vi "CR-扫码枪.vi"(8 "error in (no error)":errorcluster caption="错误输入（无错误）", 11 "名称或相对路径":string="Template Program") -> (0 "error in (no error) 2":errorcluster caption="错误输入（无错误）")   [LabVIEW 2017]
uses:
  Picture/SaveButtom.ctl
  Global System.vi
  <vilib>/Utility/xml.llb/Write to XML File(string).vi
panel:
  out "添加的路径":path
  in  "刷新":bool
  in  "测试按钮":bool
  in  "保存按钮":bool
  in  "Main":enum32{"条码获取", "测试效果 "}(tab)
  in  "扫码枪基础参数":T1 caption="参数界面"
  in  "扫码枪参数":T2={"IsNorImage"=TRUE, "Exposure Values"=100289, "ImagePath"=path "C:/Users/hedongpo/Desktop/514-hdp/Alignment Assemble System/Test Picture/B/3.bmp", "数据输出"="", "结果显示"=FALSE} caption="参数界面" {"Exposure Values" scale=0.0..200000.0}
  out "路径输出":path
  in  "Vision Paramter Save Buttom":T3
  out "system time":string
  in  "取消按钮":bool
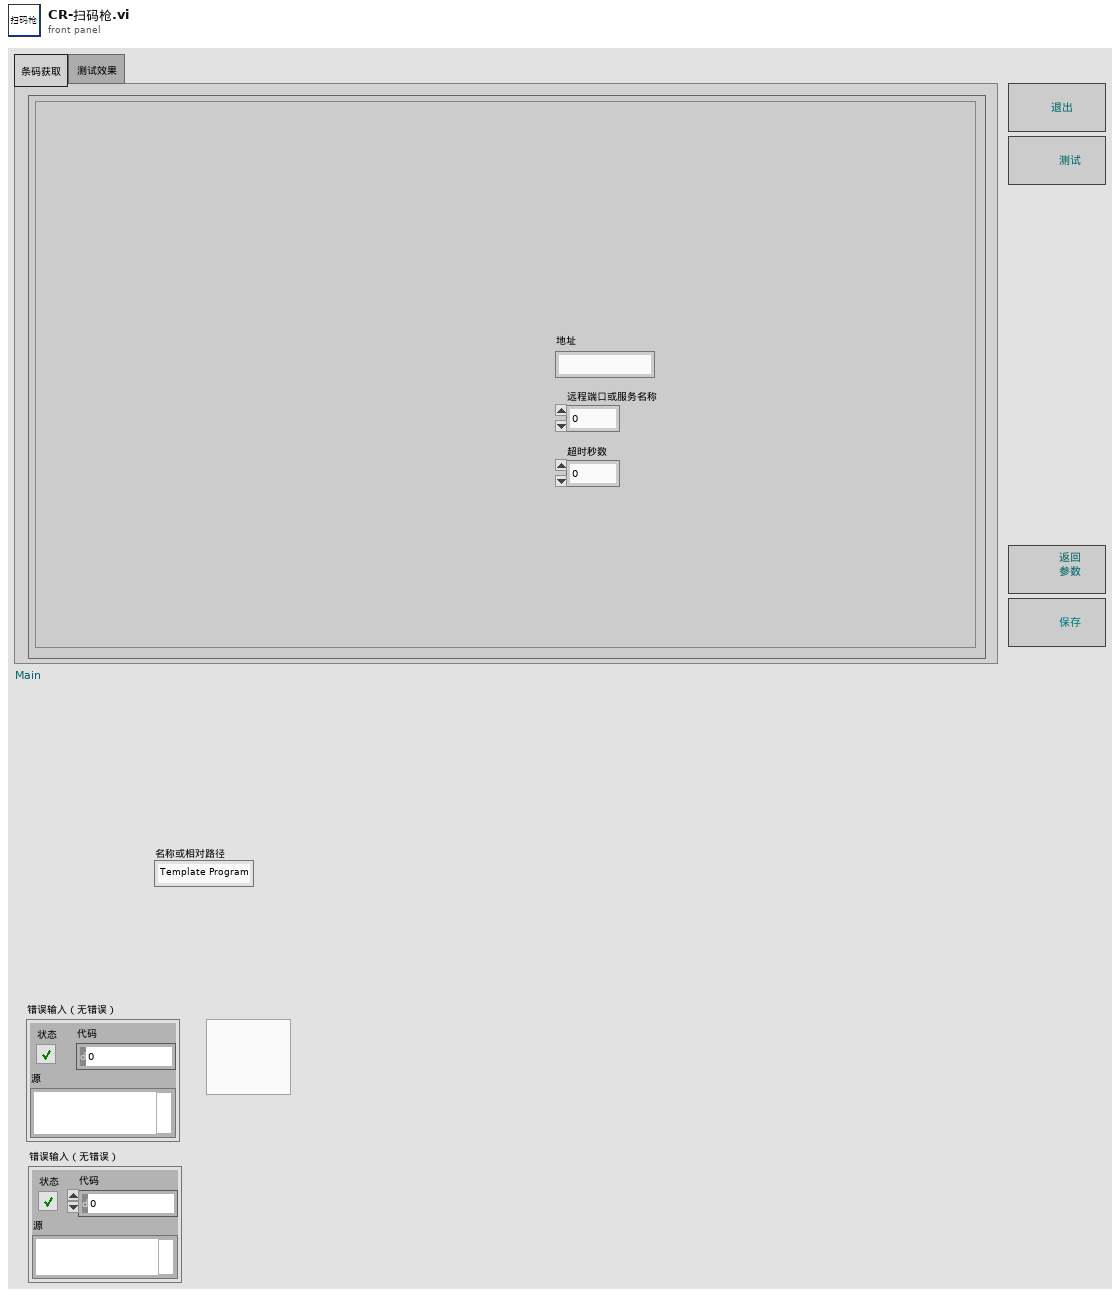
[diagram p1: front panel]
types:
  T1 = cluster{"地址":string, "远程端口或服务名称":u16, "超时秒数":dbl}
  T2 = cluster{"IsNorImage":bool, "Exposure Values":u32, "ImagePath":path, "数据输出":string, "结果显示":bool}
  T3 = typedef "SaveButtom.ctl" = bool
  T4 = cluster{"index":i32, "this vi":refnum<vi>, "error out":errorcluster}
  T5 = cluster{"master data":string, "priority":u16, "secondary data":string[]}
  T6 = cluster{"case name":string[], "queue array":refnum<queue>[]}
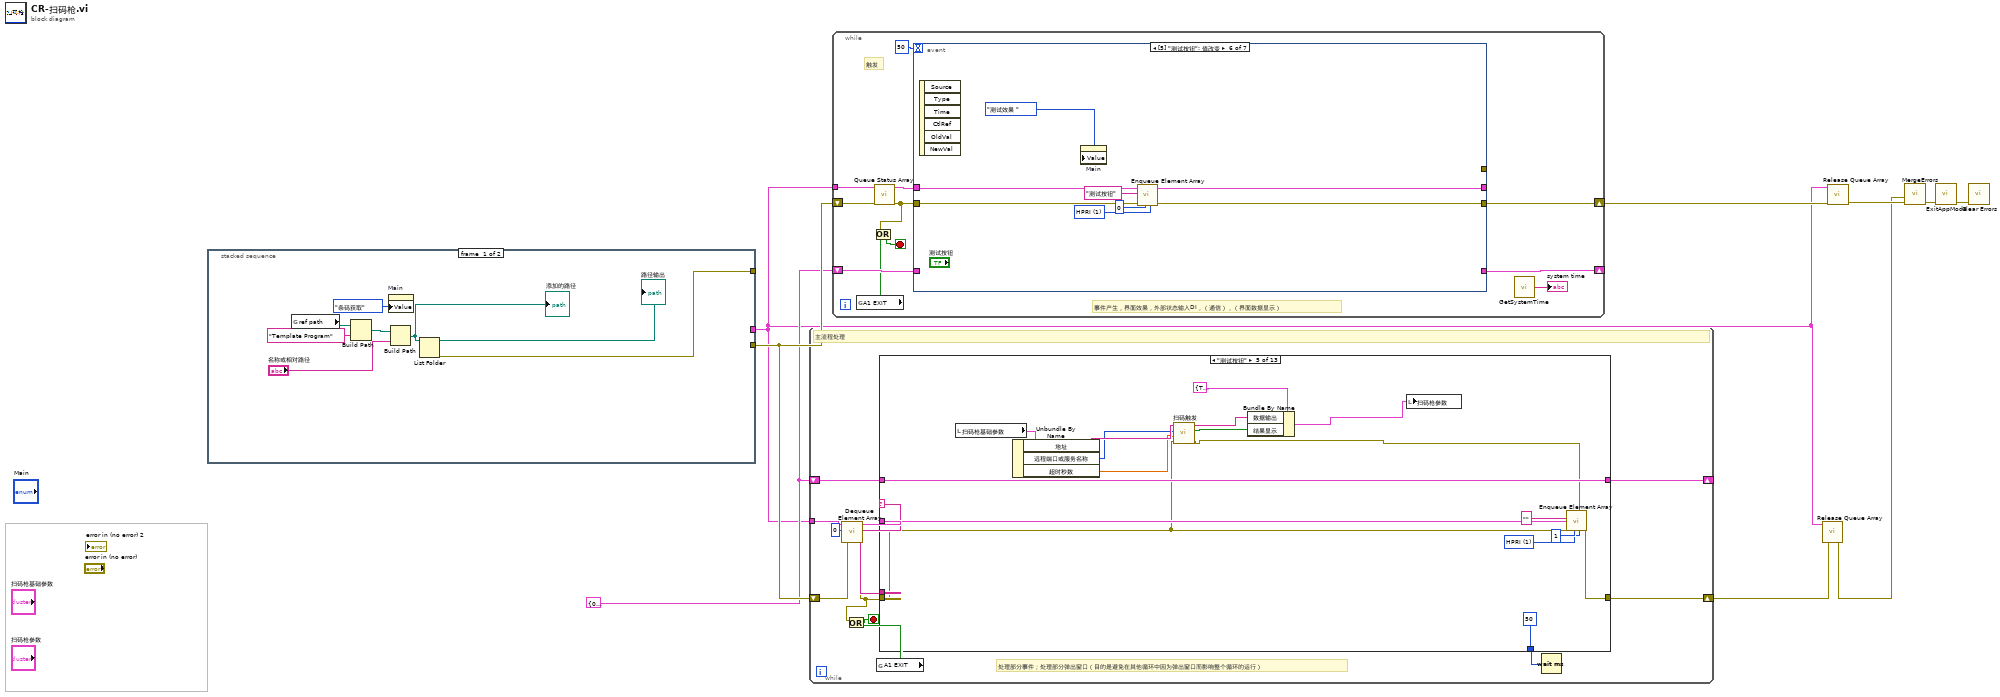
[diagram p0: block diagram]
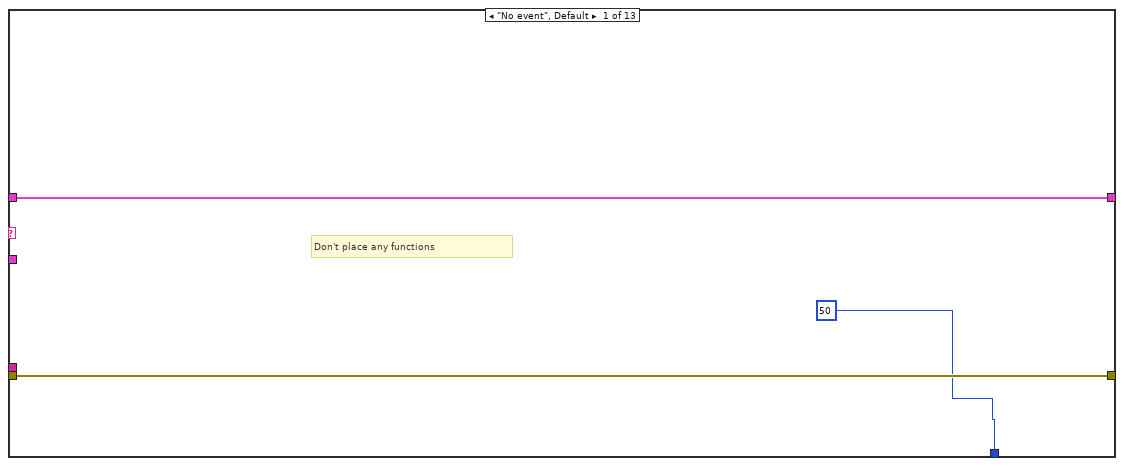
[diagram p2: hidden frame]
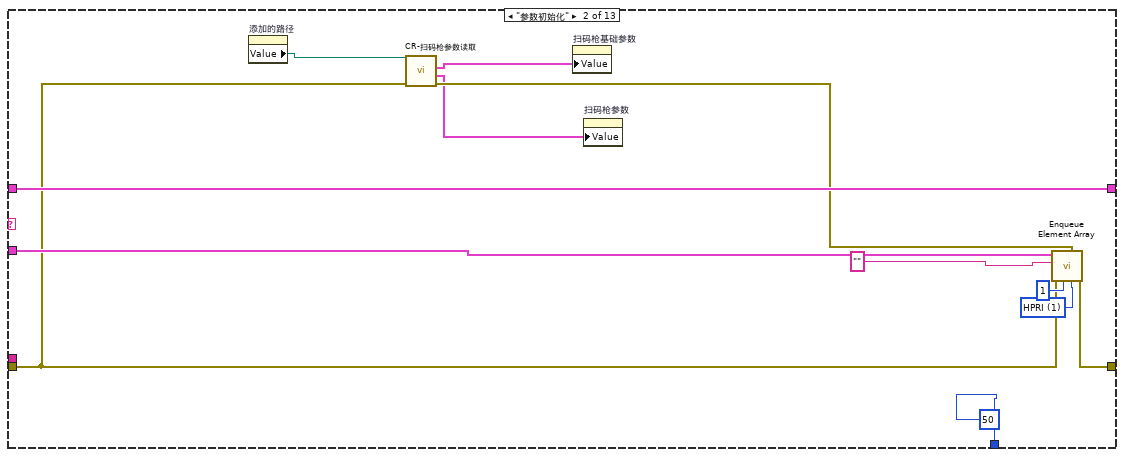
[diagram p3: hidden frame]
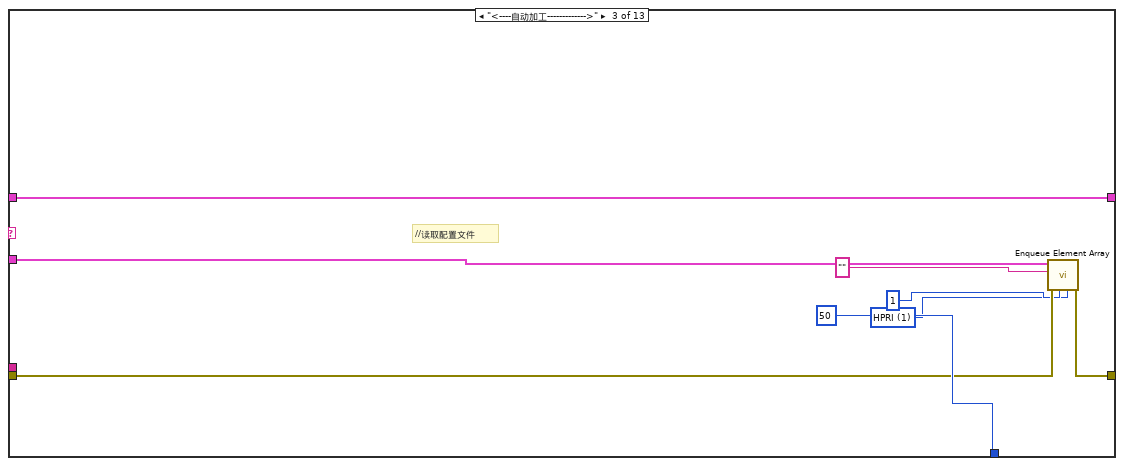
[diagram p4: hidden frame]
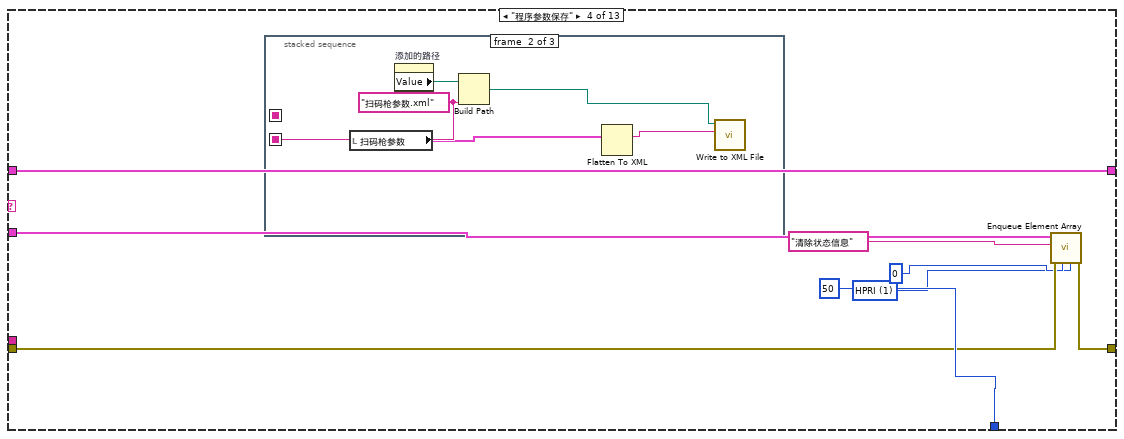
[diagram p5: hidden frame]
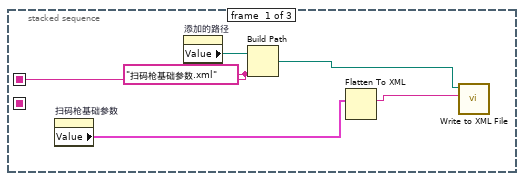
[diagram p6: hidden frame]
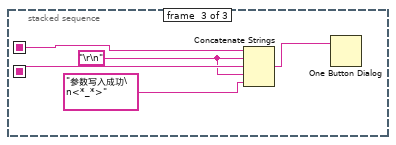
[diagram p7: hidden frame]
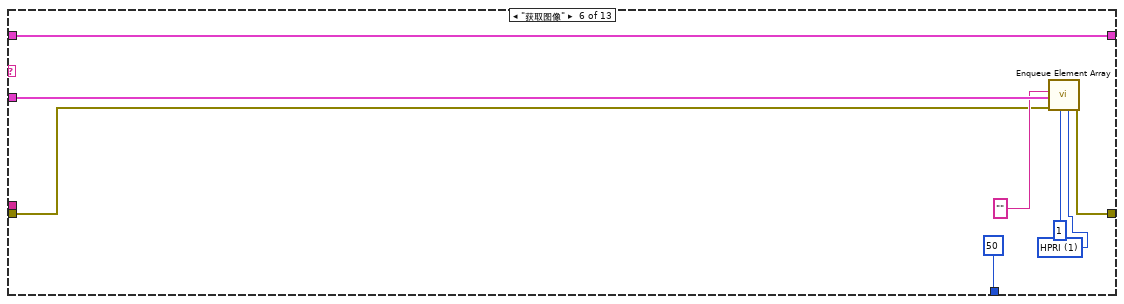
[diagram p8: hidden frame]
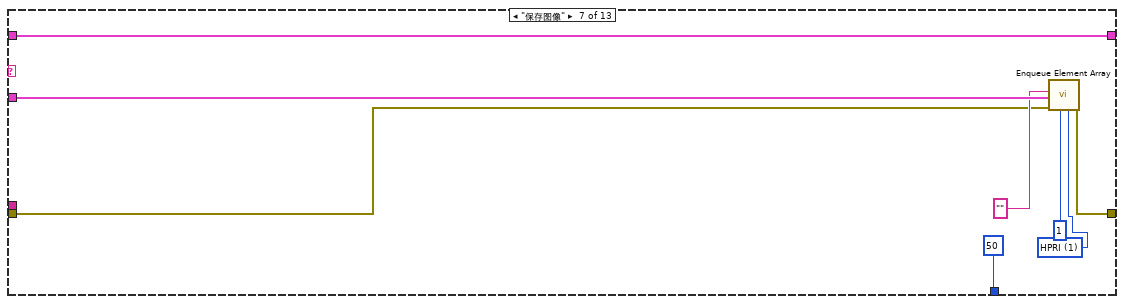
[diagram p9: hidden frame]
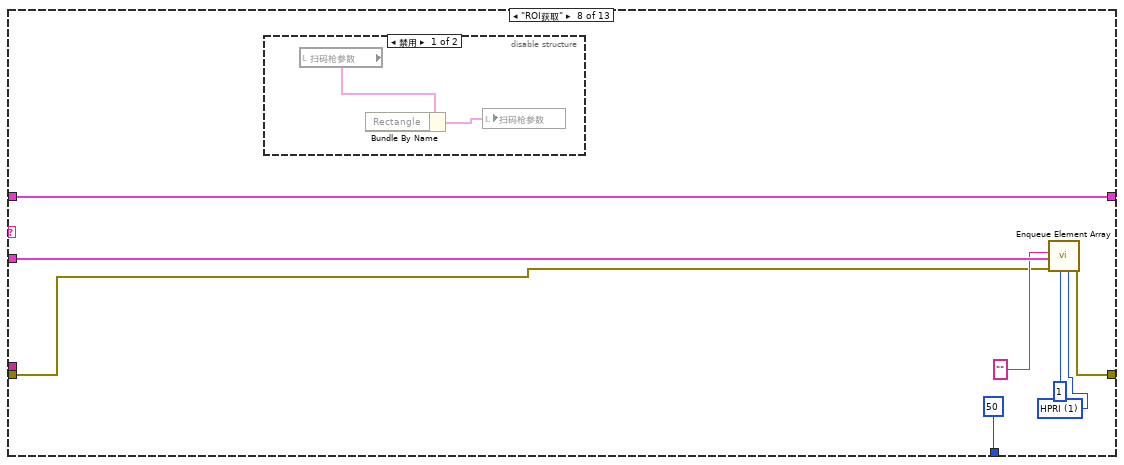
[diagram p10: hidden frame]
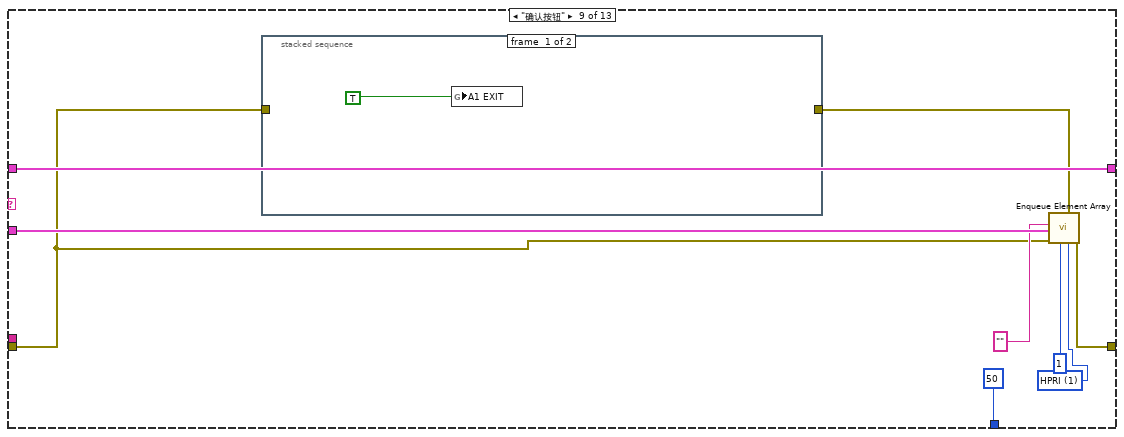
[diagram p12: hidden frame]
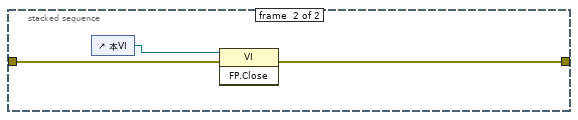
[diagram p13: hidden frame]
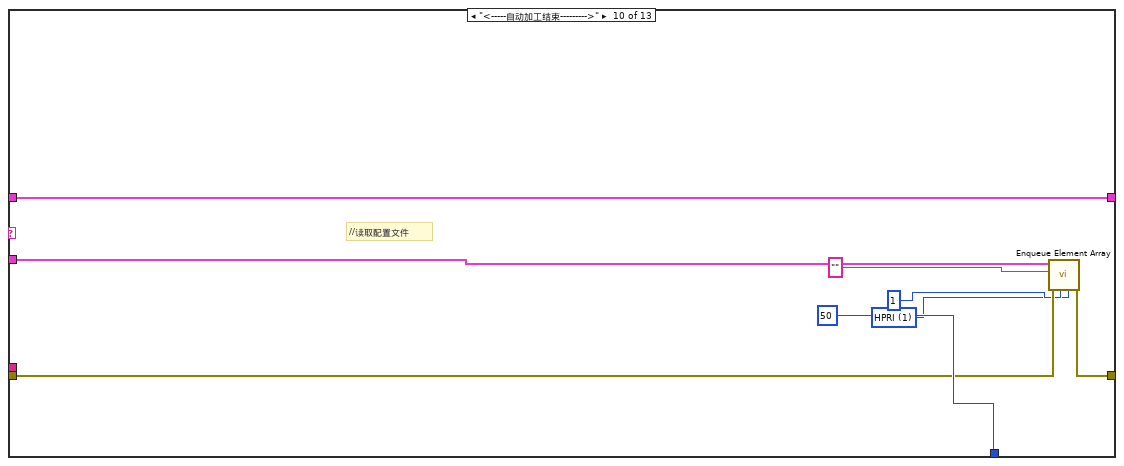
[diagram p14: hidden frame]
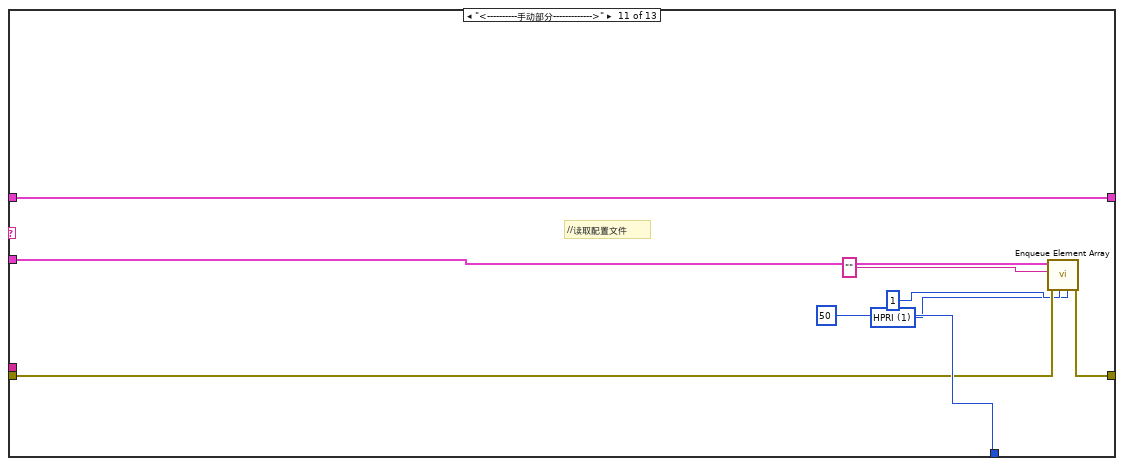
[diagram p15: hidden frame]
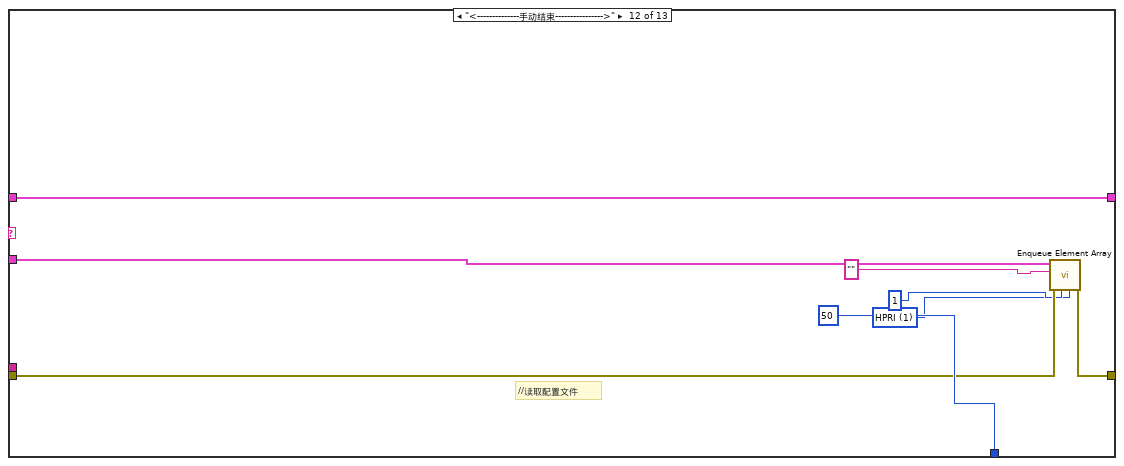
[diagram p16: hidden frame]
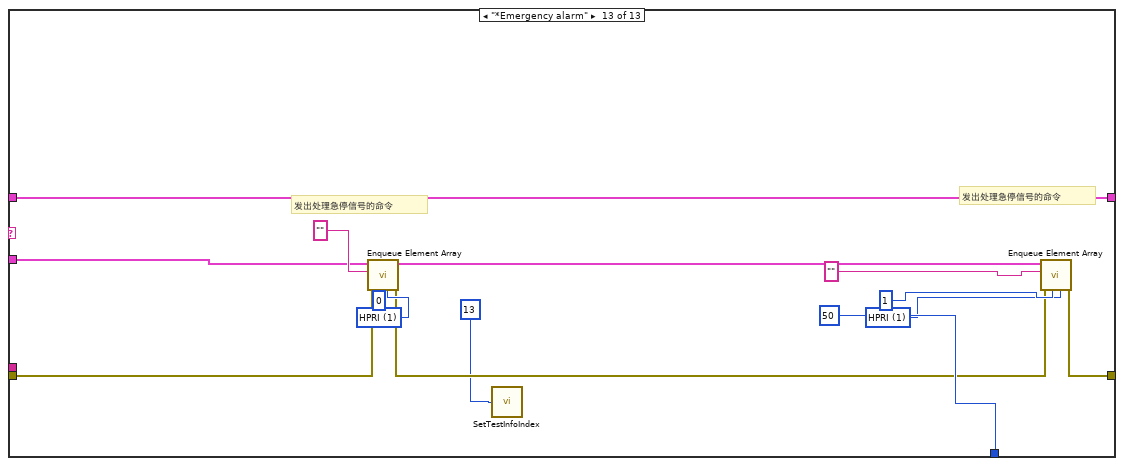
[diagram p17: hidden frame]
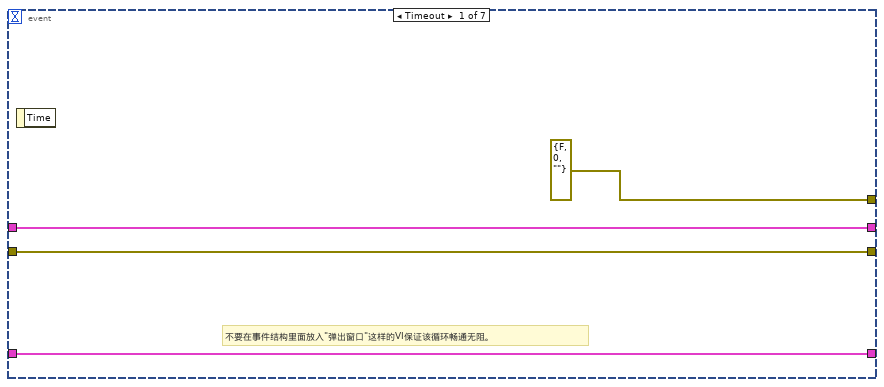
[diagram p18: hidden frame]
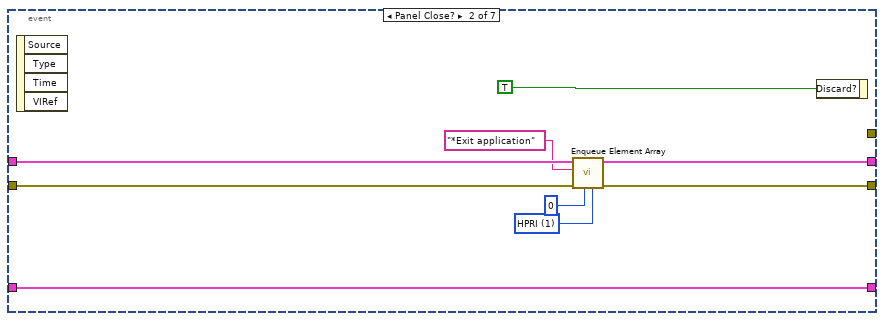
[diagram p19: hidden frame]
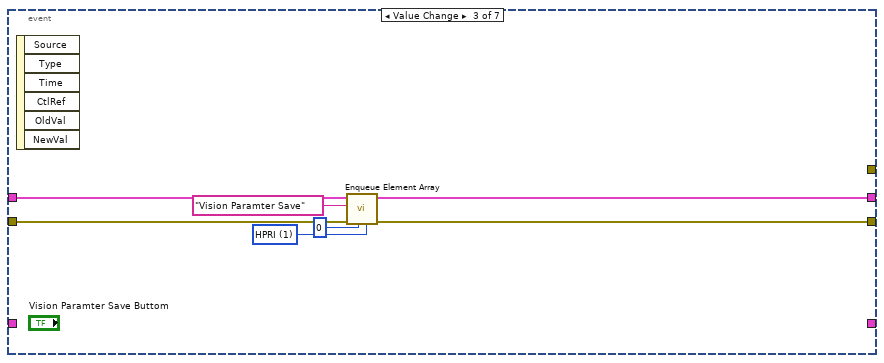
[diagram p20: hidden frame]
diagram:
  w4 = T4 {"index"=0, "this vi"=refnum, "error out"={"status"=FALSE, "code"=0, "source"=""}} ("parameter buffer")
  n1 = stacked-sequence {
    tunnel: [w15 _] -> _
    tunnel: [_ w19] -> w5
    tunnel: [_ w18] -> w1
    frame #0 {
      n2 = global read "Global System.vi" "ref path"() -> (w13:path)
      n3 = Build Path(base path=w13, name or relative path="Template Program" ("名称或相对路径")) -> (appended path=w11:path)
      n4 = property on="Main" class="TabCtl (严格)"("Value"=enum32{"条码获取", "测试效果 "}."条码获取" ("Main")) -> ()  [unwired: 2 in, 2 out]
      n5 = Build Path(base path=w11, name or relative path="名称或相对路径") -> (appended path=w17:path)
      "添加的路径" <- w17
      n6 = List Folder(path=w17) -> (path out=→"路径输出":path, error out=w15:errorcluster)  [unwired: 3 in, 2 out]
    }
    frame #1 {
      w27 = string[] ["comm queue1", "data queue 11", "data queue 12", "data queue 13", "data queue 14"]  # queue name
      w28 = 4  # queue num
      w29 = T5 {"master data"="", "priority"=0, "secondary data"=[]}  # element data type
      n7 = call "Obtain Queue Array.vi"("queue name"=w27, "element data type"=w29, "queue num"=w28) -> ("error out"=w23:errorcluster, "queue out"=w24:T6)  [unwired: 2 in, 1 out]
      n8 = call "Enqueue Element Array.vi"("queue index"=0, "error in"=w23, "master data"="参数初始化", "queue in"=w24) -> ("error out"=w22:errorcluster, "queue out"=w21:T6)  [unwired: 6 in]
      n9 = disable-structure shown="启用" {
        disable-tunnel: w22 -> [w35 w36]
        disable-tunnel: w21 -> [w34 w37]
        disable-tunnel: "Loading Variable" ("master data") -> [w33 _]
        disable-tunnel: [w31 w36] -> w19
        disable-tunnel: [w30 w37] -> w18
        frame Disabled {
          n10 = call "Enqueue Element Array.vi"("queue index"=12, "error in"=w35, "master data"=w33, "queue in"=w34) -> ("error out"=w31:errorcluster, "queue out"=w30:T6)  [unwired: 6 in]
        }
        frame Enabled {
        }
      }
    }
  }
  n11 = while {
    shift-right: [w50] -> w3
    shift-left: w5 -> [w41]
    shift-right: [w47] -> _
    shift-left: w4 -> [w48]
    tunnel: w1 -> [w43]
    stop <- w38 stop-if-true
    # "处理部分事件；处理部分弹出窗口（目的是避免在其他循环中因为弹出窗口而影响整个循环的运行）"
    # "主流程处理"
    n12 = call "Dequeue Element Array.vi"("queue in"=w43, "queue index"=0, "error in"=w41) -> ("queue out"=w46:T6, "master data"=w45:string, "secondary data"=w44:string[], "error out"=w40:errorcluster)  [unwired: 2 in, 1 out]
    n13 = global read "Global System.vi" "A1 EXIT"() -> (w39:bool)
    n14 = Or(x=w40, y=w39) -> (x .or. y?=w38:bool)
    n15 = case shown="\"测试按钮\"" w45 {
      tunnel: w46 -> [_ w64 w72 w74 w112 w120 w128 w136 w147 w159 w167 w175 w181]
      tunnel: w40 -> [w52 w57 w68 w78 w106 w114 w122 w130 w141 w155 w163 w171 w178]
      tunnel: [w52 w63 w71 w80 w111 w119 w127 w135 w146 w158 w166 w174 w189] -> w50
      tunnel: [50 50 50 50 50 50 50 50 50 50 50 50 50] -> w49
      tunnel: w48 -> [w53 w59 w69 w75 w107 w115 w123 w131 w142 w156 w164 w172 w187]
      tunnel: [w53 w59 w69 w75 w107 w115 w123 w131 w142 w156 w164 w172 w187] -> w47
      tunnel: w44 -> [_ _ _ _ _ _ _ _ _ _ _ _ _]
      frame "No event", Default {
        # "Don't place any functions"
      }
      frame "参数初始化" {
        w60 = u16 1 items=["HPRI"=1, "LPRI"=0] ("priority")
        n16 = property on="添加的路径" class="Path"() -> ("Value"=w58:path)  [unwired: 2 in, 2 out]
        n17 = call "CR-扫码枪参数读取.vi"("error in (no error)"=w57, "基路径"=w58) -> ("error out"=w56:errorcluster, "扫码枪参数"=w55:T2, "扫码枪基础参数"=w54:T1)  [unwired: 6 in]
        n18 = property on="扫码枪基础参数" class="Clust (严格)"("Value"=w54) -> ()  [unwired: 2 in, 2 out]
        n19 = property on="扫码枪参数" class="Clust (严格)"("Value"=w55) -> ()  [unwired: 2 in, 2 out]
        n20 = call "Enqueue Element Array.vi"("priority"=w60, "device error in"=w56, "queue index"=1, "error in"=w57, "master data"="" ("Element 1"), "queue in"=w64) -> ("error out"=w63:errorcluster)  [unwired: 4 in, 1 out]
      }
      frame "<----自动加工------------->" {
        w66 = u16 1 items=["HPRI"=1, "LPRI"=0] ("priority")
        # "//读取配置文件"
        n21 = call "Enqueue Element Array.vi"("priority"=w66, "queue index"=1, "error in"=w68, "master data"="" ("Element 1"), "queue in"=w72) -> ("error out"=w71:errorcluster)  [unwired: 5 in, 1 out]
      }
      frame "程序参数保存" {
        w76 = u16 1 items=["HPRI"=1, "LPRI"=0] ("priority")
        n22 = stacked-sequence {
          seq-local: [w82 _ _] -> [_ _ w95]
          seq-local: [_ w91 _] -> [_ _ w93]
          frame #0 {
            w82 = "扫码枪基础参数.xml" ("名称或相对路径")
            n23 = property on="扫码枪基础参数" class="Clust (严格)"() -> ("Value"=w85:T1)  [unwired: 2 in, 2 out]
            n24 = property on="添加的路径" class="Path"() -> ("Value"=w86:path)  [unwired: 2 in, 2 out]
            n25 = Build Path(base path=w86, name or relative path=w82) -> (appended path=w83:path)
            n26 = Flatten To XML(anything=w85) -> (xml string=w84:string)
            n27 = call-poly <vilib>:"Write to XML File.vi"("XML Input"=w84, "XML File Path"=w83) -> ()  [unwired: 7 in, 3 out]
          }
          frame #1 {
            w91 = "扫码枪参数.xml" ("名称或相对路径")
            n28 = local read "扫码枪参数"() -> (w87:T2)
            n29 = property on="添加的路径" class="Path"() -> ("Value"=w90:path)  [unwired: 2 in, 2 out]
            n30 = Build Path(base path=w90, name or relative path=w91) -> (appended path=w88:path)
            n31 = Flatten To XML(anything=w87) -> (xml string=w89:string)
            n32 = call-poly <vilib>:"Write to XML File.vi"("XML Input"=w89, "XML File Path"=w88) -> ()  [unwired: 7 in, 3 out]
          }
          frame #2 {
            w92 = "\r\n"
            n33 = Concatenate Strings(w95, w92, w93, w92, "参数写入成功\n<*_*>" ("消息")) -> (w94:string)
            n34 = One Button Dialog(message=w94) -> ()  [unwired: 1 in, 1 out]
          }
        }
        n35 = call "Enqueue Element Array.vi"("priority"=w76, "queue index"=0, "error in"=w78, "master data"="清除状态信息" ("Element 1"), "queue in"=w74) -> ("error out"=w80:errorcluster)  [unwired: 5 in, 1 out]
      }
      frame "测试按钮" {
        w108 = u16 1 items=["HPRI"=1, "LPRI"=0] ("priority")
        n36 = local read "扫码枪基础参数"() -> (w104:T1)
        n37 = Unbundle By Name(w104) -> ("地址"=w103:string, "远程端口或服务名称"=w102:u16, "超时秒数"=w97:dbl)
        n38 = call "扫码触发.vi"("error in (no error)"=w106, "超时秒数"=w97, "远程端口或服务名称"=w102, "地址"=w103) -> ("error out 2"=w105:errorcluster, "结果"=w100:bool, "数据输出"=w101:string)  [unwired: 5 in]
        n39 = Bundle By Name(cluster=T2 {"IsNorImage"=TRUE, "Exposure Values"=100289, "ImagePath"=path "C:/Users/hedongpo/Desktop/514-hdp/Alignment Assemble System/Test Picture/B/3.bmp", "数据输出"="", "结果显示"=FALSE} ("扫码枪参数"), "数据输出"=w101, "结果显示"=w100) -> (w98:T2)
        n40 = local write "扫码枪参数"(w98) -> ()
        n41 = call "Enqueue Element Array.vi"("priority"=w108, "device error in"=w105, "queue index"=1, "error in"=w106, "master data"="" ("Element 1"), "queue in"=w112) -> ("error out"=w111:errorcluster)  [unwired: 4 in, 1 out]
      }
      frame "获取图像" {
        w116 = u16 1 items=["HPRI"=1, "LPRI"=0] ("priority")
        n42 = call "Enqueue Element Array.vi"("priority"=w116, "queue index"=1, "error in"=w114, "master data"="" ("Element 1"), "queue in"=w120) -> ("error out"=w119:errorcluster)  [unwired: 5 in, 1 out]
      }
      frame "保存图像" {
        w124 = u16 1 items=["HPRI"=1, "LPRI"=0] ("priority")
        n43 = call "Enqueue Element Array.vi"("priority"=w124, "queue index"=1, "error in"=w122, "master data"="" ("Element 1"), "queue in"=w128) -> ("error out"=w127:errorcluster)  [unwired: 5 in, 1 out]
      }
      frame "ROI获取" {
        w132 = u16 1 items=["HPRI"=1, "LPRI"=0] ("priority")
        n44 = disable-structure shown="禁用" {
          frame Disabled {
            n45 = local read "扫码枪参数"() -> (w139:T2)
            n46 = Bundle By Name(cluster=w139) -> (w138:T2)  [unwired: 1 in]
            n47 = local write "扫码枪参数"(w138) -> ()
          }
          frame Enabled {
          }
        }
        n48 = call "Enqueue Element Array.vi"("priority"=w132, "queue index"=1, "error in"=w130, "master data"="" ("Element 1"), "queue in"=w136) -> ("error out"=w135:errorcluster)  [unwired: 5 in, 1 out]
      }
      frame "确认按钮" {
        w143 = u16 1 items=["HPRI"=1, "LPRI"=0] ("priority")
        n49 = stacked-sequence {
          tunnel: w141 -> [_ w151]
          tunnel: [_ w150] -> w140
          frame #0 {
            n50 = global write "Global System.vi" "A1 EXIT"(TRUE ("EXIT")) -> ()
          }
          frame #1 {
            n51 = control-ref of="本VI"() -> (w152:refnum<vi>)
            n52 = invoke class="VI" method="FP.Close"(reference=w152, error in=w151) -> (error out=w150:errorcluster)  [unwired: 1 in, 2 out]
          }
        }
        n53 = call "Enqueue Element Array.vi"("priority"=w143, "device error in"=w140, "queue index"=1, "error in"=w141, "master data"="" ("Element 1"), "queue in"=w147) -> ("error out"=w146:errorcluster)  [unwired: 4 in, 1 out]
      }
      frame "<-----自动加工结束--------->" {
        w153 = u16 1 items=["HPRI"=1, "LPRI"=0] ("priority")
        # "//读取配置文件"
        n54 = call "Enqueue Element Array.vi"("priority"=w153, "queue index"=1, "error in"=w155, "master data"="" ("Element 1"), "queue in"=w159) -> ("error out"=w158:errorcluster)  [unwired: 5 in, 1 out]
      }
      frame "<----------手动部分------------->" {
        w161 = u16 1 items=["HPRI"=1, "LPRI"=0] ("priority")
        # "//读取配置文件"
        n55 = call "Enqueue Element Array.vi"("priority"=w161, "queue index"=1, "error in"=w163, "master data"="" ("Element 1"), "queue in"=w167) -> ("error out"=w166:errorcluster)  [unwired: 5 in, 1 out]
      }
      frame "<--------------手动结束---------------->" {
        w169 = u16 1 items=["HPRI"=1, "LPRI"=0] ("priority")
        # "//读取配置文件"
        n56 = call "Enqueue Element Array.vi"("priority"=w169, "queue index"=1, "error in"=w171, "master data"="" ("Element 1"), "queue in"=w175) -> ("error out"=w174:errorcluster)  [unwired: 5 in, 1 out]
      }
      frame "*Emergency alarm" {
        w184 = u16 1 items=["HPRI"=1, "LPRI"=0] ("priority")
        w185 = u16 1 items=["HPRI"=1, "LPRI"=0] ("priority")
        # "发出处理急停信号的命令"
        # "发出处理急停信号的命令"
        n57 = call "Enqueue Element Array.vi"("priority"=w184, "queue index"=0, "error in"=w178, "master data"="" ("Element 1"), "queue in"=w181) -> ("error out"=w179:errorcluster, "queue out"=w180:T6)  [unwired: 5 in]
        n58 = call "SetTestInfoIndex.vi"("test info index"=13) -> ()
        n59 = call "Enqueue Element Array.vi"("priority"=w185, "queue index"=1, "error in"=w179, "master data"="" ("Element 1"), "queue in"=w180) -> ("error out"=w189:errorcluster)  [unwired: 5 in, 1 out]
      }
    }
    n60 = Wait (ms)(milliseconds to wait=w49) -> ()  [unwired: 1 out]
  }
  n61 = while {
    shift-right: [w194] -> w6
    shift-left: w5 -> [w198]
    shift-right: [w196] -> _
    shift-left: w4 -> [w197]
    tunnel: w1 -> [w200]
    stop <- w191 stop-if-true
    # "触发"
    # "事件产生，界面效果，外部状态输入DI，（通信），（界面数据显示）"
    n62 = global read "Global System.vi" "A1 EXIT"() -> (w192:bool)
    n63 = call "Queue Status Array.vi"("error in (no error)"=w198, "queue in"=w200) -> ("error out"=w193:errorcluster, "queue out"=w195:T6)  [unwired: 4 in]
    n64 = Or(x=w193, y=w192) -> (x .or. y?=w191:bool)
    n65 = event shown="[5] \"测试按钮\": 值改变" {
      selector: _ -> [_ _ _ _ _ _ _]
      dyn-events: _ -> [_ _ _ _ _ _ _]
      timeout: 50 -> [_ _ _ _ _ _ _]
      tunnel: w197 -> [w205 w213 _ _ _ _ _]
      tunnel: [w205 w213 _ _ _ _ _] -> w196
      tunnel: [errorcluster {"status"=FALSE, "code"=0, "source"=""} ("error out") _ _ _ _ _ _] -> _
      tunnel: w195 -> [w203 w212 w218 w225 w232 w240 w247]
      tunnel: w193 -> [w202 w211 w217 w224 w231 w239 w246]
      tunnel: [w202 w210 w215 w222 w229 w237 w244] -> w194
      tunnel: [w203 w209 w216 w223 w230 w238 w245] -> _
      event Timeout {
        # "不要在事件结构里面放入\"弹出窗口\"这样的VI保证该循环畅通无阻。"
        n66 = event-data() -> ()  [unwired: 1 in, 1 out]
      }
      event Panel Close? {
        w207 = u16 1 items=["HPRI"=1, "LPRI"=0] ("priority")
        n67 = event-data() -> ()  [unwired: 1 in, 4 out]
        n68 = call "Enqueue Element Array.vi"("priority"=w207, "queue index"=0, "error in"=w211, "master data"="*Exit application", "queue in"=w212) -> ("error out"=w210:errorcluster, "queue out"=w209:T6)  [unwired: 5 in]
        n69 = event-data("Discard?"=TRUE) -> ()  [unwired: 1 in, 1 out]
      }
      event Value Change {
        w220 = u16 1 items=["HPRI"=1, "LPRI"=0] ("priority")
        n70 = event-data() -> ()  [unwired: 1 in, 6 out]
        n71 = call "Enqueue Element Array.vi"("priority"=w220, "queue index"=0, "error in"=w217, "master data"="Vision Paramter Save", "queue in"=w218) -> ("error out"=w215:errorcluster, "queue out"=w216:T6)  [unwired: 5 in]
      }
      event "取消按钮": Value Change {
        w227 = u16 1 items=["HPRI"=1, "LPRI"=0] ("priority")
        n72 = event-data() -> ()  [unwired: 1 in, 6 out]
        n73 = call "Enqueue Element Array.vi"("priority"=w227, "queue index"=0, "error in"=w224, "master data"="确认按钮", "queue in"=w225) -> ("error out"=w222:errorcluster, "queue out"=w223:T6)  [unwired: 5 in]
      }
      event "保存按钮": Value Change {
        w234 = u16 1 items=["HPRI"=1, "LPRI"=0] ("priority")
        n74 = event-data() -> ()  [unwired: 1 in, 6 out]
        n75 = call "Enqueue Element Array.vi"("priority"=w234, "queue index"=0, "error in"=w231, "master data"="程序参数保存", "queue in"=w232) -> ("error out"=w229:errorcluster, "queue out"=w230:T6)  [unwired: 5 in]
      }
      event "测试按钮": Value Change {
        w242 = u16 1 items=["HPRI"=1, "LPRI"=0] ("priority")
        n76 = event-data() -> ()  [unwired: 1 in, 6 out]
        n77 = property on="Main" class="TabCtl (严格)"("Value"=enum32{"条码获取", "测试效果 "}."测试效果 " ("Main")) -> ()  [unwired: 2 in, 2 out]
        n78 = call "Enqueue Element Array.vi"("priority"=w242, "queue index"=0, "error in"=w239, "master data"="测试按钮", "queue in"=w240) -> ("error out"=w237:errorcluster, "queue out"=w238:T6)  [unwired: 5 in]
      }
      event "刷新": Value Change {
        n79 = event-data() -> ()  [unwired: 1 in, 6 out]
        n80 = disable-structure shown="禁用" {
          disable-tunnel: w247 -> [w251 _]
          disable-tunnel: w246 -> [w250 _]
          disable-tunnel: [w249 _] -> w245
          disable-tunnel: [w248 _] -> w244
          frame Disabled {
            w253 = u16 1 items=["HPRI"=1, "LPRI"=0] ("priority")
            # "刷新"
            n81 = call "Enqueue Element Array.vi"("priority"=w253, "queue index"=0, "error in"=w250, "master data"="刷新", "queue in"=w251) -> ("error out"=w248:errorcluster, "queue out"=w249:T6)  [unwired: 5 in]
          }
          frame Enabled {
          }
        }
      }
    }
    n82 = call "GetSystemTime.vi"() -> ("date/time string"=→"system time":string)  [unwired: 7 in]
  }
  n83 = call "Release Queue Array.vi"("error in"=w3, "queue in"=w1) -> ("error out"=w2:errorcluster)  [unwired: 2 in, 3 out]
  n84 = call "Release Queue Array.vi"("error in"=w6, "queue in"=w1) -> ("error out"=w9:errorcluster)  [unwired: 2 in, 3 out]
  n85 = call "MergeErrors.vi"("error in 3 (no error)"=w2, "error in 4 (no error)"=w9) -> ("error out"=w8:errorcluster)  [unwired: 6 in]
  n86 = call "ExitAppMode.vi"("error in (no error)"=w8) -> ("error out"=w7:errorcluster)  [unwired: 10 in]
  n87 = call <vilib>:"Clear Errors.vi"("error in (no error)"=w7) -> ()  [unwired: 5 in, 2 out]
